vi "DatetimeToSQLDT1.vi"(10 "input string":string) -> (2 "resulting string":string)   [LabVIEW 2012]
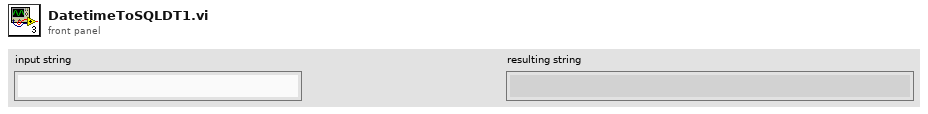
[diagram p1: front panel]
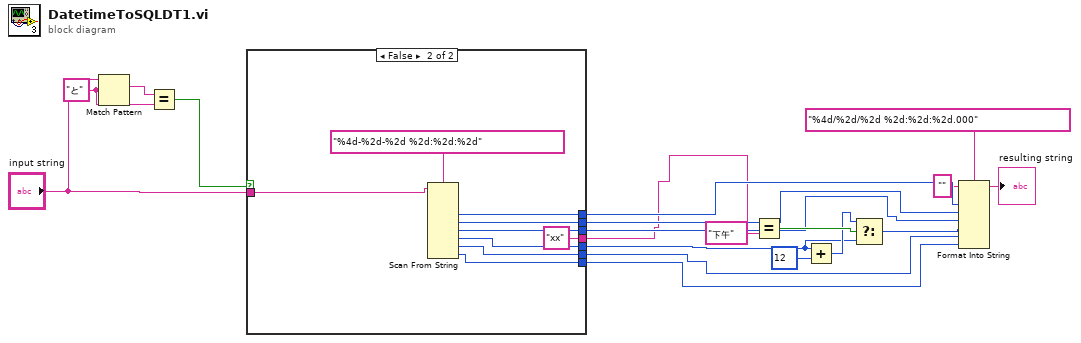
[diagram p0: block diagram]
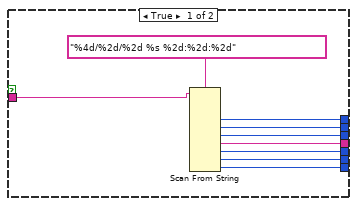
[diagram p2: hidden frame]
diagram:
  w2 = "と" ("regular expression")
  n1 = Match Pattern(string="input string", regular expression=w2) -> (match substring=w3:string)  [unwired: 1 in, 3 out]
  n2 = Equal?(x=w3, y=w2) -> (x = y?=w1:bool)
  n3 = case shown="False" w1 {
    tunnel: [w27 w32] -> w15
    tunnel: [w26 w36] -> w14
    tunnel: [w25 w35] -> w13
    tunnel: [w24 w34] -> w12
    tunnel: [w23 w31] -> w10
    tunnel: [w22 w30] -> w9
    tunnel: "input string" -> [w21 w33]
    tunnel: [w20 "xx"] -> w5
    frame True {
      n4 = Scan From String(format string="%4d/%2d/%2d %s %2d:%2d:%2d", input string=w21) -> (output 1=w26:i32, output 2=w25:i32, output 3=w24:i32, output 4=w20:string, output 5=w27:i32, output 6=w23:i32, output 7=w22:i32)  [unwired: 9 in, 3 out]
    }
    frame False {
      n5 = Scan From String(format string="%4d-%2d-%2d %2d:%2d:%2d", input string=w33) -> (output 1=w36:i32, output 2=w35:i32, output 3=w34:i32, output 4=w32:i32, output 5=w31:i32, output 6=w30:i32)  [unwired: 8 in, 3 out]
    }
  }
  n6 = Equal?(x=w5, y="下午") -> (x = y?=w17:bool)
  n7 = Add(x=w15, y=12) -> (x+y=w16:i32)
  n8 = Select(t=w16, s=w17, f=w15) -> (s? t:f=w11:i32)
  n9 = Format Into String(format string="%4d/%2d/%2d %2d:%2d:%2d.000", initial string="", w14, w13, w12, w11, w10, w9) -> (resulting string=→"resulting string":string)  [unwired: 1 in, 1 out]
